vi "View_noise.vi"() -> ()   [LabVIEW 2015]
uses:
  <vilib>/FPGAPlugInAG/PXIe-7971R/niLvFpga_Open_PXIe-7971R.vi
  <vilib>/Utility/error.llb/Error Cluster From Error Code.vi
  Program Files (x86)/National Instruments/LabVIEW 2015/Targets/NI/FPGA/StockFPGA_IntfPrivate/ScriptTemplates/StockFPGA_PlugInRead32.vi
  <vilib>/rvi/errors/niLvFpgaAdjustHostInterfaceError.vi
  <vilib>/FPGAPlugInAG/PXIe-7971R/niLvFpga_Close_PXIe-7971R.vi
  <vilib>/rvi/interface/nirviOpenFPGA/nirviOpenFPGA.xnode
  FPGA Bitfiles/FPGAnew_FPGATarget_Graphdetnoise_Kx9imQGLZRE.lvbitx
  <vilib>/rvi/interface/nirviReadWriteControl/nirviReadWriteControl.xnode
  <vilib>/rvi/interface/nirviCloseFPGA/nirviCloseFPGA.xnode
  NiFpgaLv.dll
  <vilib>/FPGAPlugInAG/PXIe-7971R/niLvFpga_Read32_PXIe-7971R.vi
  <vilib>/rvi/interface/nirviReadWriteControl/niFpgaRWControlAccessTimeoutTemplate.vi
  <vilib>/rvi/errors/niLvFpgaMergeErrorWithErrorCode.vi
panel:
  out "det3":i16[](graph)
  out "det 2":i32[](graph)
  out "XY Graph 2":cluster{"time":u32[], "Det 2":i16[]}(graph)
  out "XY Graph":cluster{"Det 1":i16[], "time":u32[]}(graph)
  in  "time":u32[](array[numeric])
  out "Det 1":i16[](array[numeric])
  out "Corr 2":i32(graph)
  out "Corr 1":i32[](array[numeric])
  out "Corr 2":i32[](array[numeric])
  out "Corr 1":i32(graph)
  out "loop count":u32
  out "Det 2":i16[](array[numeric])
  in  "stop":bool
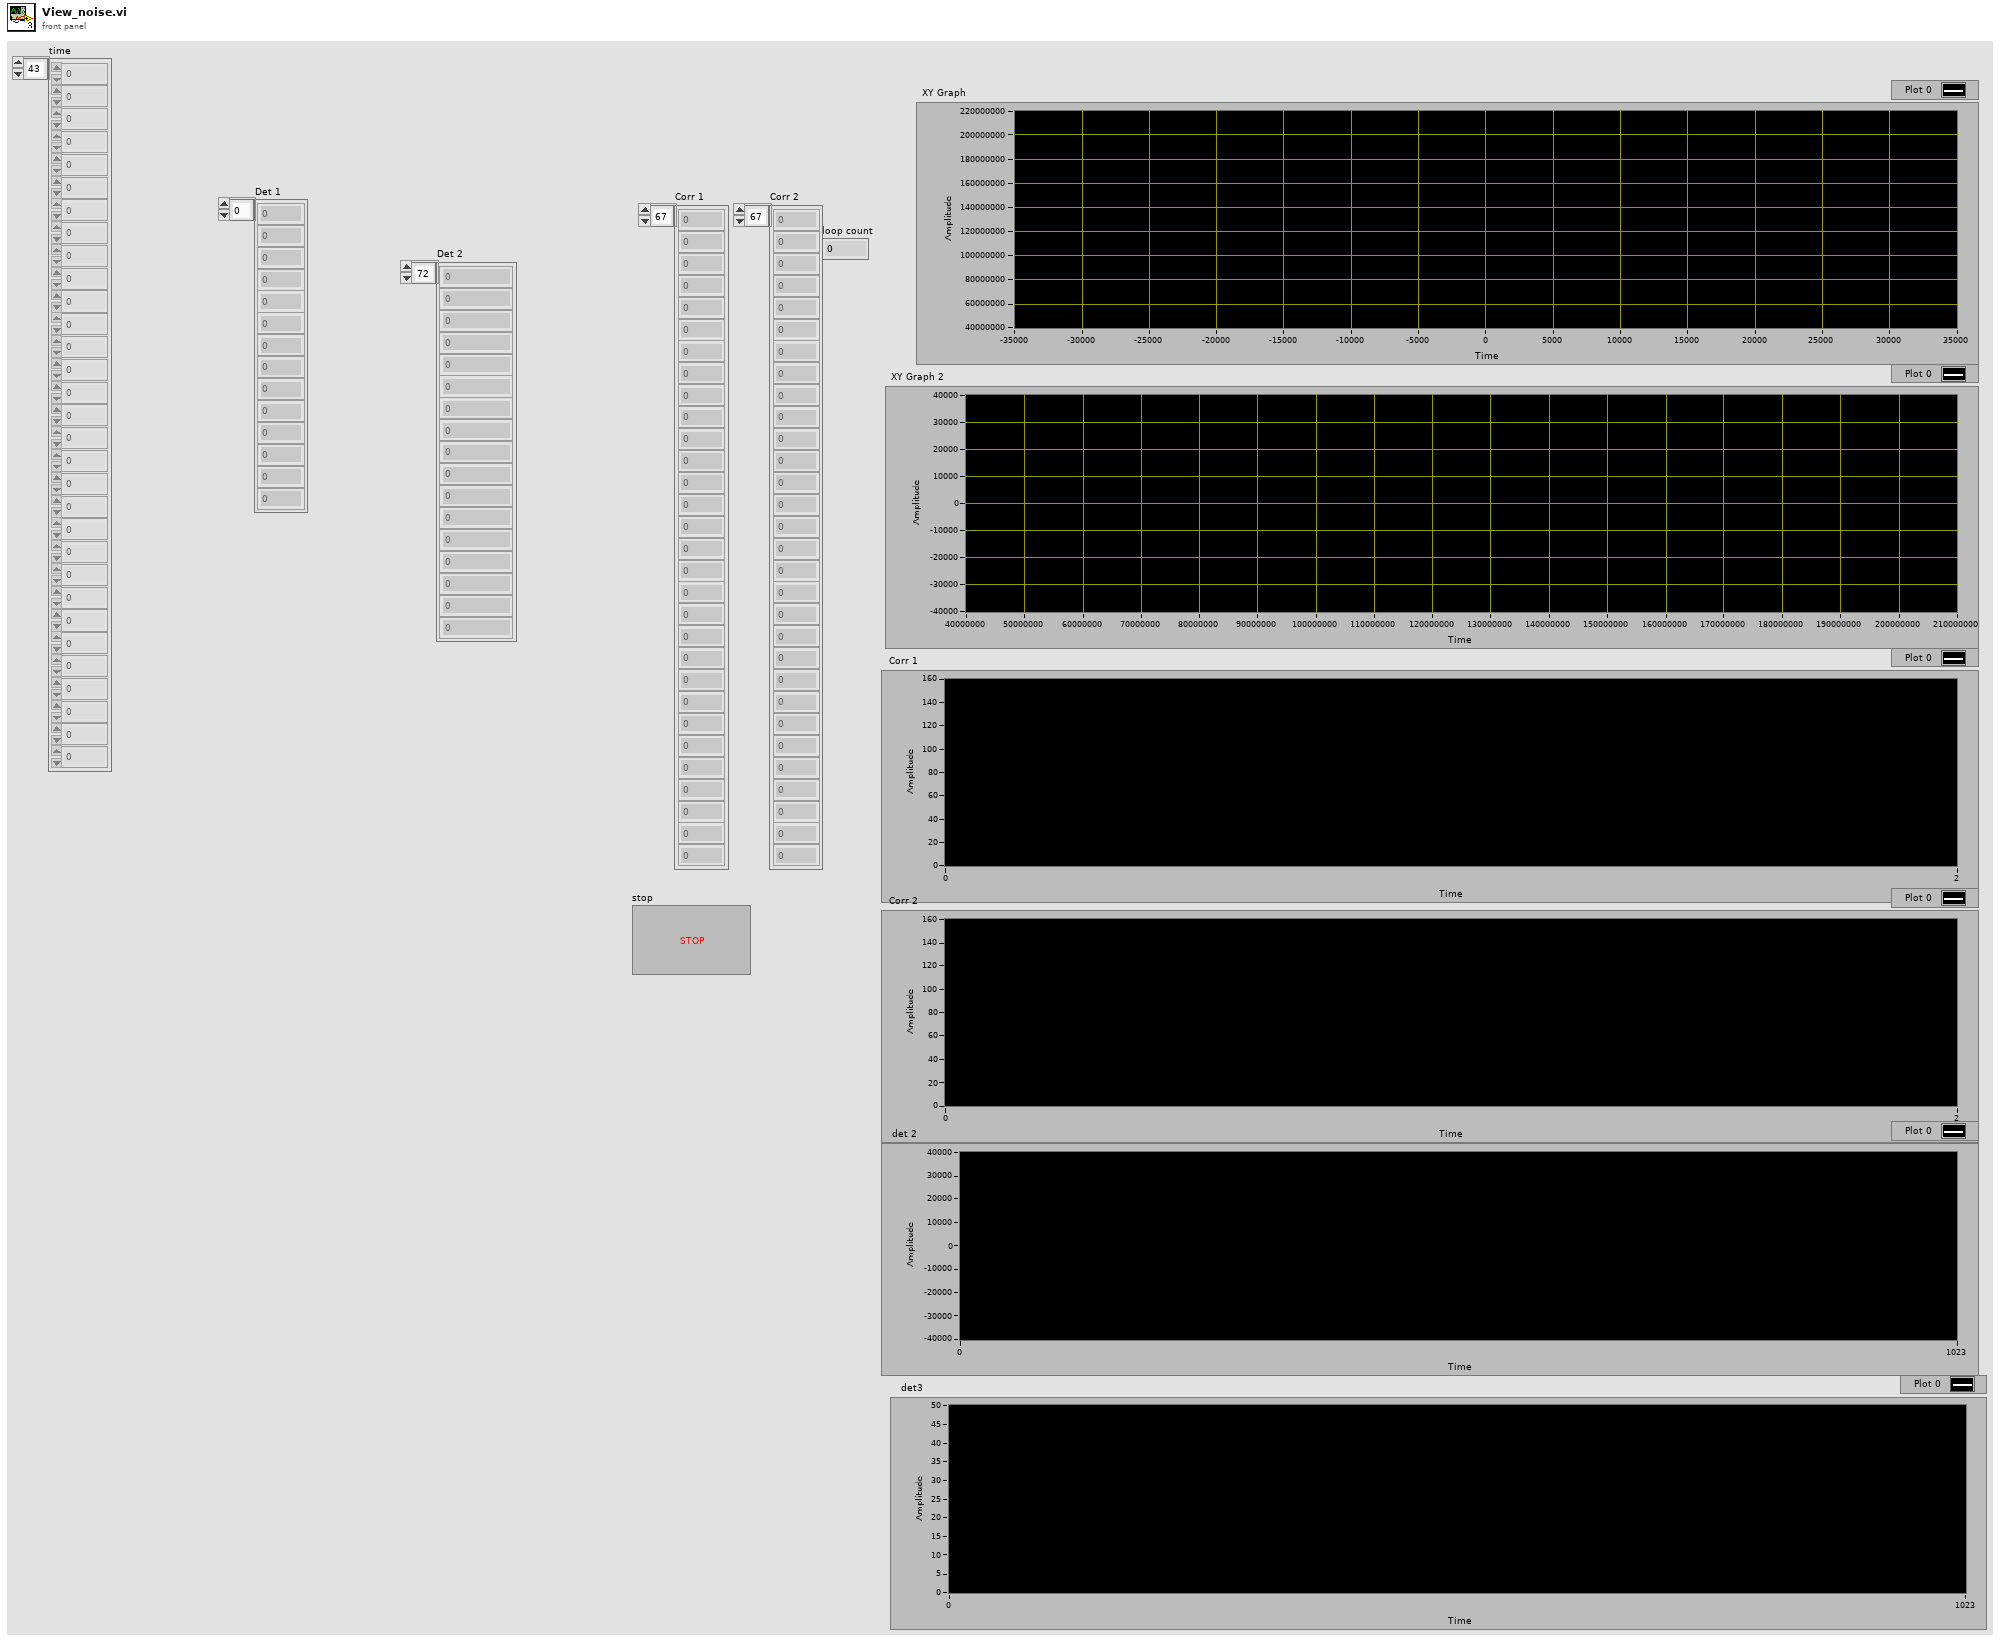
[diagram p1: front panel]
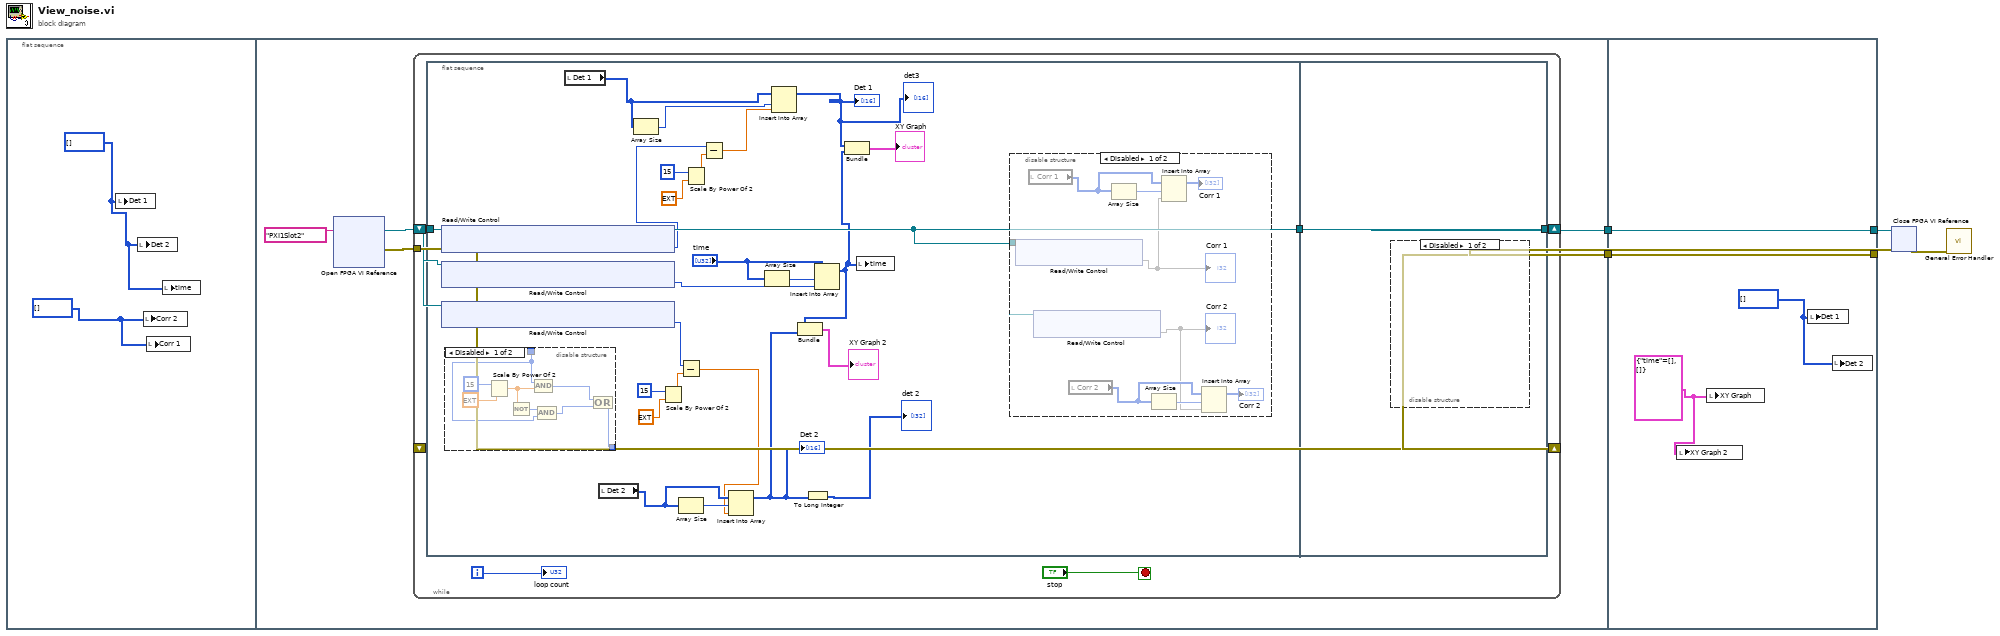
[diagram p0: block diagram]
diagram:
  n1 = flat-sequence {
    tunnel: [w10] -> w2
    tunnel: [w8] -> w1
    tunnel: [w64] -> w4
    tunnel: [w65] -> w5
    tunnel: w2 -> [w65]
    tunnel: w1 -> [w64]
    frame #0 {
      w7 = i32[] []
      w6 = i16[] []
      n2 = local write "Det 1"(w6) -> ()
      n3 = local write "Det 2"(w6) -> ()
      n4 = local write "Corr 2"(w7) -> ()
      n5 = local write "Corr 1"(w7) -> ()
      n6 = local write "time"(w6) -> ()
    }
    frame #1 {
      n7 = xnode "Open FPGA VI Reference"("resource name"=tag "PXI1Slot2") -> ("FPGA VI Reference Out"=w11:refnum<k20>, "error out"=w9:errorcluster)  [unwired: 1 in]
      n8 = while {
        shift-right: [w16] -> w10
        shift-left: w11 -> [w14]
        tunnel: w9 -> [w15]
        shift-right: [w15] -> w8
        shift-left: _ -> [_]
        i -> [w17]
        stop <- "stop" stop-if-true
        n9 = flat-sequence {
          tunnel: w14 -> [w41]
          tunnel: [w42] -> w13
          tunnel: [w61] -> w16
          tunnel: w13 -> [w61]
          frame #0 {
            n10 = xnode "Read/Write Control"("FPGA VI Reference In"=w41) -> ("FPGA VI Reference Out"=w42:refnum<k20>, "IO Module\\AI 2"=w19:u16)  [unwired: 1 in, 1 out]
            n11 = xnode "Read/Write Control"("FPGA VI Reference In"=w41) -> ("IO Module\\AI 3"=w28:u16)  [unwired: 1 in, 2 out]
            n12 = xnode "Read/Write Control"("FPGA VI Reference In"=w41) -> ("Tick Count(uSec)"=w39:u32)  [unwired: 1 in, 2 out]
            n13 = disable-structure shown="Disabled" {
              disable-tunnel: [w47 _] -> _
              disable-tunnel: _ -> [w46 _]
              frame Disabled {
                n14 = Scale By Power Of 2(n=i16 15, x=ext 1.0) -> (x*2^n=w49:ext)
                n15 = Not(x=w49) -> (.not. x?=w48:u32)
                n16 = Compound Arithmetic op=AND(w46, w49) -> (w45:i32)
                n17 = Compound Arithmetic op=AND(w48, w46) -> (w44:u32)
                n18 = Compound Arithmetic op=OR(w45, w44) -> (w47:u32)
              }
              frame Enabled {
              }
            }
            n19 = local read "Det 1"() -> (w38:i16[])
            n20 = local read "Det 2"() -> (w43:i16[])
            n21 = Array Size(array=w38) -> (size(s)=w37:i32)
            n22 = Scale By Power Of 2(n=i16 15, x=ext 1.0) -> (x*2^n=w27:ext)
            n23 = Subtract(x=w28, y=w27) -> (x-y=w26:ext)
            n24 = Array Size(array=w43) -> (size(s)=w35:i32)
            n25 = Scale By Power Of 2(n=i16 15, x=ext 1.0) -> (x*2^n=w21:ext)
            n26 = Subtract(x=w19, y=w21) -> (x-y=w20:ext)
            n27 = Insert Into Array(array=w43, index=w35, new element=w26) -> (w24:i16[])
            "Det 2" <- w24
            n28 = Array Size(array="time") -> (size(s)=w40:i32)
            n29 = Insert Into Array(array=w38, index=w37, new element=w20) -> (w31:i16[])
            "Det 1" <- w31
            "det3" <- w31
            n30 = To Long Integer(number=w24) -> (32bit integer=→"det 2":i32[])
            n31 = Insert Into Array(array="time", index=w40, new element=w39) -> (w32:u32[])
            n32 = Bundle("time"=w32, "Det 2"=w24) -> (→"XY Graph 2":cluster{"time":u32[], "Det 2":i16[]})  [unwired: 1 in]
            n33 = Bundle("Det 1"=w31, "time"=w32) -> (→"XY Graph":cluster{"Det 1":i16[], "time":u32[]})  [unwired: 1 in]
            n34 = local write "time"(w32) -> ()
            n35 = disable-structure shown="Disabled" {
              disable-tunnel: w42 -> [w60 _]
              frame Disabled {
                n36 = xnode "Read/Write Control"("FPGA VI Reference In"=w60) -> ("Detector 1 Correlation Out"=w52)  [unwired: 1 in, 2 out]
                "Corr 1" <- w52
                n37 = local read "Corr 1"() -> (w53:i32[])
                n38 = xnode "Read/Write Control"("FPGA VI Reference In"=w60) -> ("Detector 3 Correlation Out"=w56)  [unwired: 1 in, 2 out]
                "Corr 2" <- w56
                n39 = local read "Corr 2"() -> (w59:i32[])
                n40 = Array Size(array=w53) -> (size(s)=w55:i32)
                n41 = Array Size(array=w59) -> (size(s)=w57:i32)
                n42 = Insert Into Array(array=w53, index=w55, new element=w52) -> (→"Corr 1":i32[])
                n43 = Insert Into Array(array=w59, index=w57, new element=w56) -> (→"Corr 2":i32[])
              }
              frame Enabled {
              }
            }
          }
          frame #1 {
            n44 = disable-structure shown="Disabled" {
              frame Disabled {
              }
              frame Enabled {
              }
            }
          }
        }
        "loop count" <- w17
      }
    }
    frame #2 {
      w62 = cluster{"time":i16[], i16[]} {"time"=[], []} ("XY Graph")
      w63 = i16[] []
      n45 = local write "XY Graph 2"(w62) -> ()
      n46 = local write "XY Graph"(w62) -> ()
      n47 = local write "Det 1"(w63) -> ()
      n48 = local write "Det 2"(w63) -> ()
    }
  }
  n49 = xnode "Close FPGA VI Reference"("FPGA VI Reference In"=w5, "error in"=w4) -> ("error out"=w3:errorcluster)
  n50 = call <vilib>:"General Error Handler.vi"("error in (no error)"=w3) -> ()  [unwired: 10 in, 5 out]
